vi "RT Driver VI.vi"(7 "Operation":T1, 11 "Device Reference in":T2 format="%.0x") -> (0 "Error Code":i32)   [LabVIEW 2020, in "PXI-2512 Engine.lvlib"]
uses:
  PXI-2512 Engine.lvlib
  <vilib>/NI/NIVS Inline Async API/_VS Inline Async API/VS Inline Async API/VS Inline Async API.lvclass
  <vilib>/NI VeriStand/Custom Device API/Custom Device API.lvlib
  <vilib>/NI VeriStand/Custom Device Tools/Custom Device Utility Library/Custom Device Utility Library.lvlib
  Shared/Compiled.Settings.ctl
  Shared/PXI-2512 Shared.lvlib
  Shared/Constants.vi
  PXI-2512.Async.vi
  <vilib>/NI VeriStand/Custom Device API/Get Item Property (Variant).vi
  <vilib>/NI VeriStand/Custom Device API/Custom Device Item Ref.ctl
  <vilib>/NI VeriStand/Custom Device API/Hardware Interface Driver VI Operation.ctl
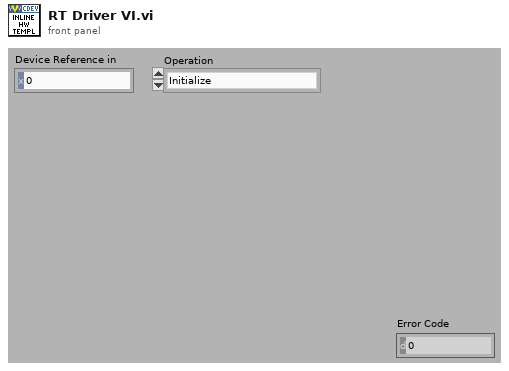
[diagram p1: front panel]
types:
  T1 = typedef "Custom Device API.lvlib/Hardware Interface Driver VI Operation.ctl" = enum16{"Initialize", "Start", "Read Data from HW", "Write Data to HW", "Close"}
  T2 = typedef "Custom Device API.lvlib/Custom Device Item Ref.ctl" = u64
  T3 = typedef "PXI-2512 Shared.lvlib/Compiled.Settings.ctl" = cluster{"Name":string, "Async Init Timeout":u16, "Hardware Device Name":string}
  T4 = cluster{"Async":refnum<class "VS Inline Async API.lvclass">, "Compiled.Settings":T3}
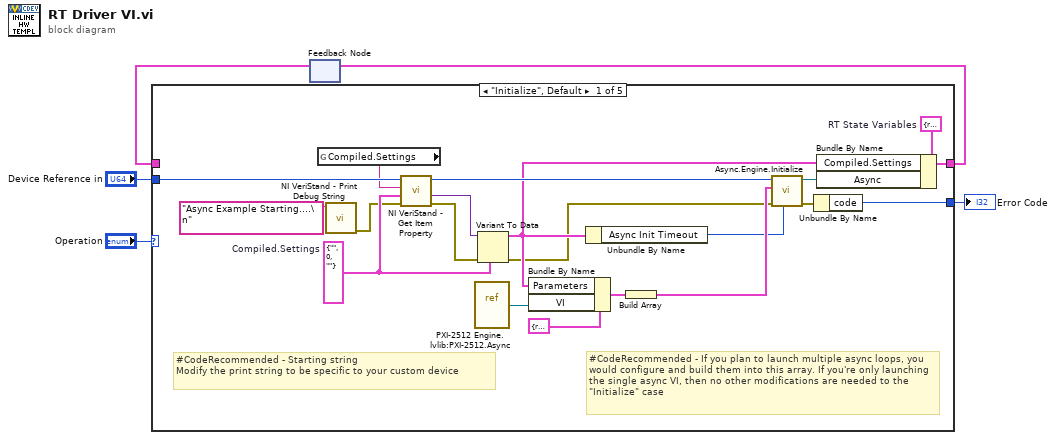
[diagram p0: block diagram]
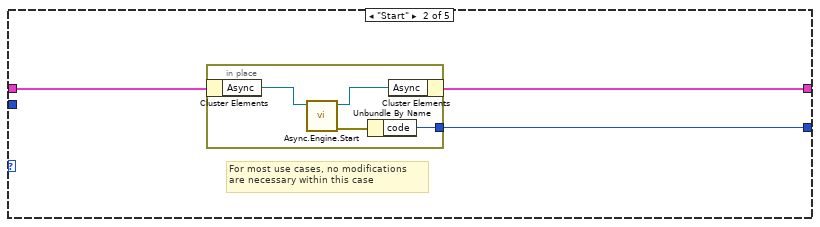
[diagram p2: hidden frame]
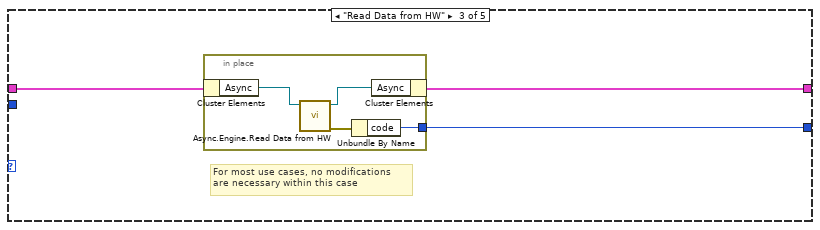
[diagram p3: hidden frame]
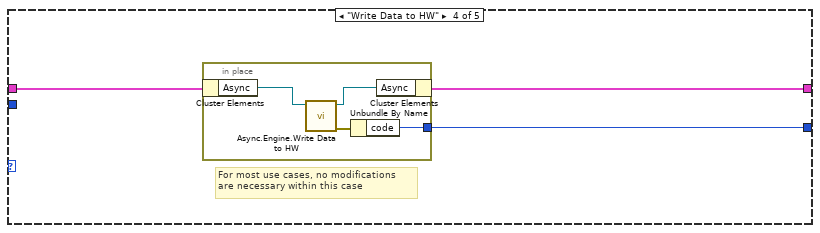
[diagram p4: hidden frame]
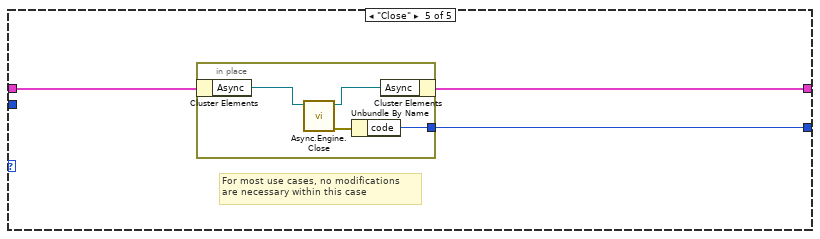
[diagram p5: hidden frame]
diagram:
  n1 = feedback #1() -> (w3:T4)  [unwired: 1 out]
  n2 = case shown="\"Initialize\", Default" "Operation" {
    tunnel: [w23 w27 w33 w40 w48] -> w4
    tunnel: w3 -> [_ w28 w35 w41 w49]
    tunnel: "Device Reference in" -> [w20 _ _ _ _]
    tunnel: [w25 w26 w34 w42 w47] -> w1
    frame "Initialize", Default {
      w15 = T4 {"Async"=refnum, "Compiled.Settings"={"Name"="", "Async Init Timeout"=0, "Hardware Device Name"=""}}  # RT State Variables
      w16 = T3 {"Name"="", "Async Init Timeout"=0, "Hardware Device Name"=""}  # Compiled.Settings
      # "#CodeRecommended - Starting string\nModify the print string to be specific to your custom device"
      # "#CodeRecommended - If you plan to launch multiple async loops, you would configure and build them into this array. If you're only launching the single async VI, then no other modifications are needed to the \"Initialize\" case"
      n3 = global read "Constants.vi" "Compiled.Settings"() -> (w17:string)
      n4 = call <vilib>:"NI VeriStand - Print Debug String.vi"("Message"="Async Example Starting....\n") -> ("error out"=w12:errorcluster)  [unwired: 10 in]
      n5 = call-poly <vilib>:"NI VeriStand - Get Item Property.vi"("error in (no error)"=w12, "Default Value"=w16, "Property Name"=w17, "Item Ref in"=w20) -> ("error out"=w19:errorcluster, "Value"=w18:variant, "Item Ref out"=w13:T2)  [unwired: 4 in, 1 out]
      n6 = vi-ref "PXI-2512 Engine.lvlib:PXI-2512.Async.vi"() -> (w10:refnum<vi>)
      n7 = Variant To Data(error in=w19, type=w16, Variant=w18) -> (data=w9:T3, error out=w7:errorcluster)
      n8 = Bundle By Name(cluster=cluster{"VI":refnum<vi>, "Parameters":variant} {"VI"=refnum, "Parameters"=variant} ("Process"), "Parameters"=w9, "VI"=w10) -> (w21:cluster{"VI":refnum<vi>, "Parameters":variant})
      n9 = Unbundle By Name(w9) -> ("Async Init Timeout"=w8:u16)
      n10 = Build Array(w21) -> (w14:cluster{"VI":refnum<vi>, "Parameters":variant}[])
      n11 = call <vilib>:"Async.Engine.Initialize.vi"("Timeout (ms) (5000)"=w8, "error in (no error)"=w7, "Processes"=w14, "Custom Device Ref"=w13) -> ("error out"=w6:errorcluster, "Async"=w24:refnum<class "VS Inline Async API.lvclass">)  [unwired: 6 in]
      n12 = Unbundle By Name(w6) -> ("code"=w25:i32)
      n13 = Bundle By Name(cluster=w15, "Compiled.Settings"=w9, "Async"=w24) -> (w23:T4)
    }
    frame "Start" {
      # "For most use cases, no modifications \nare necessary within this case"
      n14 = in-place {
        in-place-border: [w29] -> w26
        n15 = in-place-cluster #2(w28) -> ("Async"=w32:refnum<class "VS Inline Async API.lvclass">)
        n16 = call <vilib>:"Async.Engine.Start.vi"("VS Inline Async API in"=w32) -> ("error out"=w30:errorcluster, "VS Inline Async API out"=w31:refnum<class "VS Inline Async API.lvclass">)  [unwired: 9 in]
        n17 = Unbundle By Name(w30) -> ("code"=w29:i32)
        n18 = in-place-cluster #2("Async"=w31) -> (w27:T4)
      }
    }
    frame "Read Data from HW" {
      # "For most use cases, no modifications \nare necessary within this case"
      n19 = in-place {
        in-place-border: [w37] -> w34
        n20 = in-place-cluster #3(w35) -> ("Async"=w39:refnum<class "VS Inline Async API.lvclass">)
        n21 = call <vilib>:"Async.Engine.Read Data from HW.vi"("Async in"=w39) -> ("error out"=w36:errorcluster, "Async out"=w38:refnum<class "VS Inline Async API.lvclass">)  [unwired: 9 in]
        n22 = Unbundle By Name(w36) -> ("code"=w37:i32)
        n23 = in-place-cluster #3("Async"=w38) -> (w33:T4)
      }
    }
    frame "Write Data to HW" {
      # "For most use cases, no modifications \nare necessary within this case"
      n24 = in-place {
        in-place-border: [w46] -> w42
        n25 = in-place-cluster #4(w41) -> ("Async"=w44:refnum<class "VS Inline Async API.lvclass">)
        n26 = call <vilib>:"Async.Engine.Write Data to HW.vi"("VS Inline Async API in"=w44) -> ("error out"=w45:errorcluster, "VS Inline Async API out"=w43:refnum<class "VS Inline Async API.lvclass">)  [unwired: 9 in]
        n27 = Unbundle By Name(w45) -> ("code"=w46:i32)
        n28 = in-place-cluster #4("Async"=w43) -> (w40:T4)
      }
    }
    frame "Close" {
      # "For most use cases, no modifications \nare necessary within this case"
      n29 = in-place {
        in-place-border: [w51] -> w47
        n30 = in-place-cluster #5(w49) -> ("Async"=w53:refnum<class "VS Inline Async API.lvclass">)
        n31 = call <vilib>:"Async.Engine.Close.vi"("Async in"=w53) -> ("error out"=w50:errorcluster, "Async out"=w52:refnum<class "VS Inline Async API.lvclass">)  [unwired: 9 in]
        n32 = Unbundle By Name(w50) -> ("code"=w51:i32)
        n33 = in-place-cluster #5("Async"=w52) -> (w48:T4)
      }
    }
  }
  "Error Code" <- w1
  n34 = feedback-in #1(w4) -> ()
